vi "Auton Script Builder.vi"(11 "Export?":bool) -> ()   [LabVIEW 2015]
uses:
  Robot Global Data.vi
  <vilib>/Utility/file.llb/Read Delimited Spreadsheet (DBL).vi
  <vilib>/Utility/file.llb/Write Delimited Spreadsheet (DBL).vi
panel:
  out "error out 2":errorcluster
  out "error out":errorcluster
  out "Export Successful?":bool
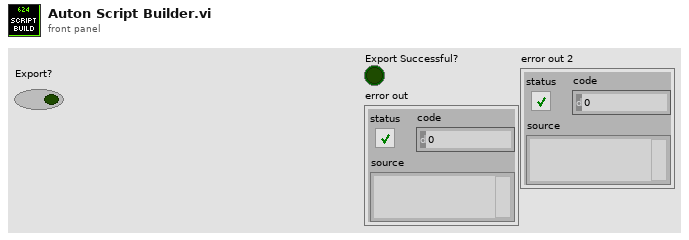
[diagram p1: front panel]
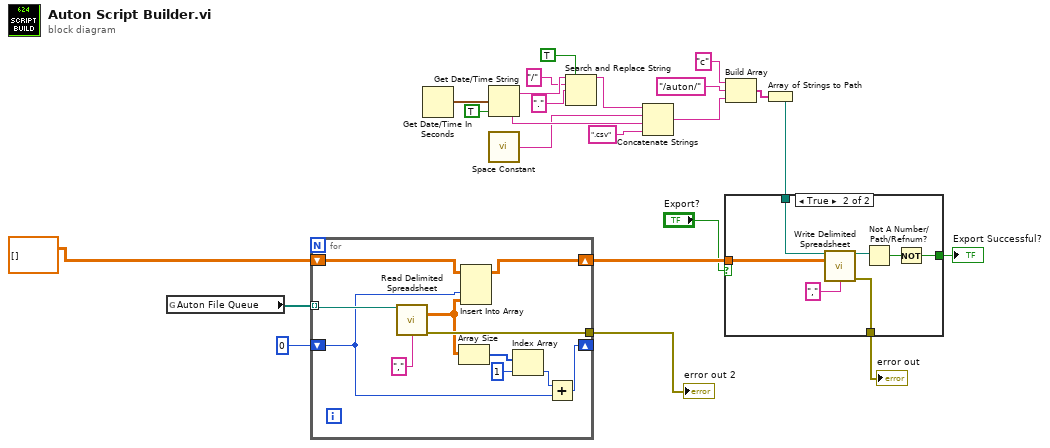
[diagram p0: block diagram]
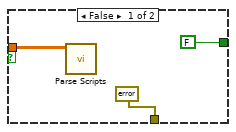
[diagram p2: hidden frame]
diagram:
  n1 = global read "Robot Global Data.vi" "Auton File Queue"() -> (w8:path[])
  n2 = for {
    tunnel: w8 -> [w34] mode=indexing
    shift-right: [w32] -> w22
    shift-left: dbl[][] [] -> [w33]
    tunnel: [w30] -> w10
    shift-right: [w25] -> _
    shift-left: 0 -> [w24]
    n3 = call-poly <vilib>:"Read Delimited Spreadsheet.vi"("file path (dialog if empty)"=w34, "delimiter (\\t)"="," ("delimiter (\\t)")) -> ("all rows"=w29:dbl[][], "error out"=w30:errorcluster)  [unwired: 8 in, 4 out]
    n4 = Array Size(array=w29) -> (size(s)=w28:i32[])
    n5 = Insert Into Array(array=w33, index (col)=w24, new element=w29) -> (w32:dbl[][])  [unwired: 1 in]
    n6 = Index Array(array=w28, index=1) -> (element=w26:i32)
    n7 = Add(x=w26, y=w24) -> (x+y=w25:i32)
  }
  "error out 2" <- w10
  n8 = Get Date/Time In Seconds() -> (seconds since 1Jan1904=w15:timestamp)
  n9 = Get Date/Time String(seconds (now)=w15, want seconds? (F)=TRUE) -> (date string=w6:string, time string=w13:string)  [unwired: 1 in]
  n10 = call <vilib>:"Space Constant.vi"() -> ("String"=w1:string)
  n11 = Search and Replace String(replace all?=TRUE ("replace all? (F)"), input string=w6, search string="/", replace string="." ("replace string (\"\")")) -> (result string=w2:string)  [unwired: 4 in, 3 out]
  n12 = Concatenate Strings(w2, w1, w13, ".csv" ("element")) -> (w11:string)
  n13 = Build Array("c", "/auton/", w11) -> (w18:string[])
  n14 = Array of Strings to Path(0:w18) -> (2:w17:path)  [unwired: 1 in]
  n15 = case shown="True" "Export?" {
    tunnel: w22 -> [w37 w44]
    tunnel: w17 -> [_ w43]
    tunnel: [FALSE w39] -> w16
    tunnel: [errorcluster {"status"=FALSE, "code"=0, "source"=""} ("error out") w38] -> w9
    frame False {
      n16 = call "Parse Scripts.vi"("Array"=w37) -> ()  [unwired: 11 in]
    }
    frame True {
      n17 = call-poly <vilib>:"Write Delimited Spreadsheet.vi"("file path (dialog if empty)"=w43, "2D data"=w44, "delimiter (\\t)"="," ("delimiter (\\t)")) -> ("new file path (Not A Path if cancelled)"=w41:path, "error out"=w38:errorcluster)  [unwired: 11 in]
      n18 = Not A Number/Path/Refnum?(number/path/refnum=w41) -> (NaN/Path/Refnum?=w40:bool)
      n19 = Not(x=w40) -> (.not. x?=w39:bool)
    }
  }
  "Export Successful?" <- w16
  "error out" <- w9
